vi "ChoreoRatio.vi"(7 "Traj Pos Points":cluster{"x":dbl, "y":dbl, "th":dbl}[](array[cluster]), 8 "Path Type":T1, 9 "dt array":dbl[](array[numeric]), 10 "Path Points":cluster{"x":dbl, "y":dbl}[](array[cluster]), 11 "Path Type":T2) -> (2 "Choreo path?":bool, 3 "Output Ratio":dbl)   [LabVIEW 2025]
uses:
  Types/Path Type.ctl
  Types/Segment Type.ctl
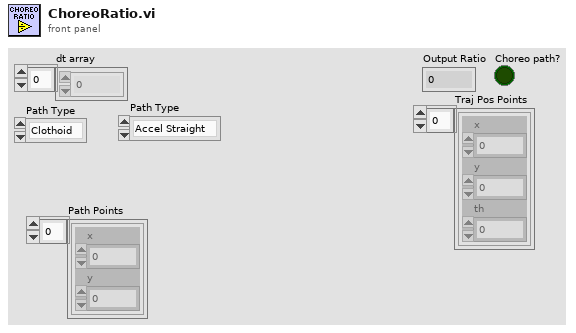
[diagram p1: front panel]
types:
  T1 = typedef "Segment Type.ctl" = enum16{"Accel Straight", "Const Straight", "Blend", "Circle", "Bezier", "Choreo"}
  T2 = typedef "Path Type.ctl" = enum16{"Clothoid", "Bezier", "Choreo"}
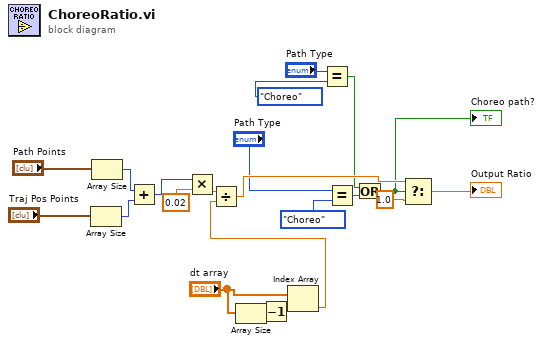
[diagram p0: block diagram]
diagram:
  n1 = Array Size(array="Traj Pos Points") -> (size(s)=w3:i32)
  n2 = Array Size(array="Path Points") -> (size(s)=w4:i32)
  n3 = Add(x=w4, y=w3) -> (x+y=w2:i32)
  n4 = Multiply(x=w2, y=0.02) -> (x*y=w18:dbl)
  n5 = Array Size(array="dt array") -> (size(s)=w16:i32)
  n6 = Decrement(x=w16) -> (x-1=w15:i32)
  n7 = Index Array(array="dt array", index=w15) -> (element=w14:dbl)
  n8 = Divide(x=w18, y=w14) -> (x/y=w13:dbl)
  n9 = Equal?(x="Path Type", y=Segment_Type."Choreo") -> (x = y?=w6:bool)
  n10 = Equal?(x="Path Type", y=Path_Type."Choreo") -> (x = y?=w9:bool)
  n11 = Or(x=w6, y=w9) -> (x .or. y?=w1:bool)
  "Choreo path?" <- w1
  n12 = Select(t=w13, s=w1, f=1.0) -> (s? t:f=→"Output Ratio":dbl)
